vi "SLSC Add Channel Features.vi"(4 "Cluster Enum":T2, 5 "Documentation":string, 6 "description-en":string, 7 "SLSCChannelPath":string, 8 "error in (no error)":errorcluster, 9 "documentation-en":string, 10 "SLSC Command Name":string, 11 "Channel Ref":T1 format="%.0x") -> (0 "error out":errorcluster, 3 "Channel Ref Out":T1 format="%.0x")   [LabVIEW 2015, in "SLSC CD System Explorer.lvlib"]
doc: "Set the channel properties based on the SLSC information, description and documentation."
uses:
  SLSC CD System Explorer.lvlib
  <vilib>/NI Veristand/Custom Device API/Custom Device Item Ref.ctl
  <vilib>/NI Veristand/Custom Device API/Set Item Property (String).vi
  <vilib>/NI VeriStand/Custom Device API/Custom Device API.lvlib
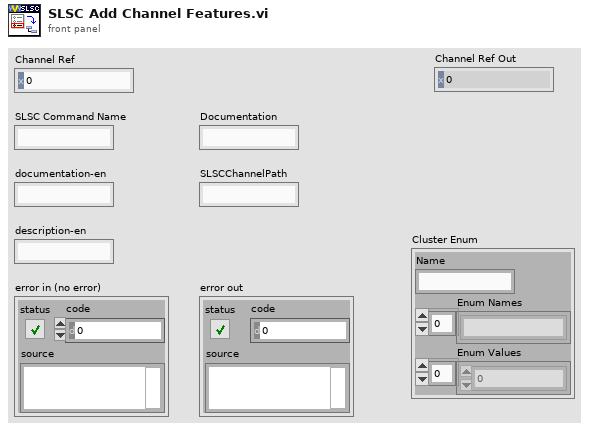
[diagram p1: front panel]
types:
  T1 = typedef "Custom Device API.lvlib/Custom Device Item Ref.ctl" = u64
  T2 = cluster{"Name":string, "Enum Names":string[], "Enum Values":i32[]}
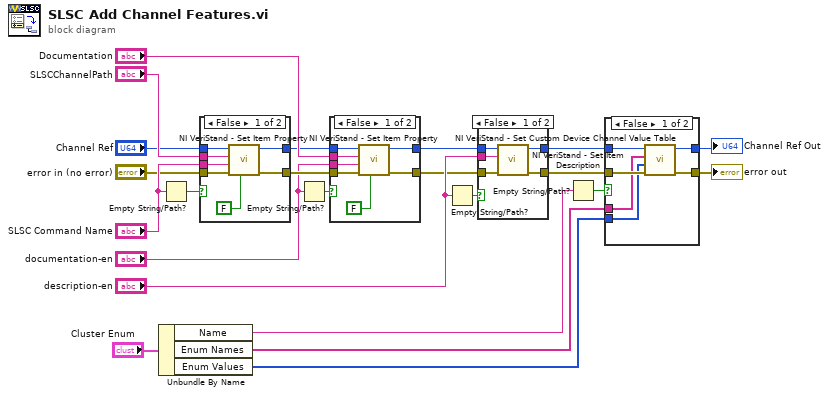
[diagram p0: block diagram]
diagram:
  n1 = Unbundle By Name("Cluster Enum") -> ("Name"=w2:string, "Enum Names"=w4:string[], "Enum Values"=w3:i32[])
  n2 = Empty String/Path?(string/path="SLSC Command Name") -> (empty?=w15:bool)
  n3 = case shown="False" w15 {
    tunnel: "Channel Ref" -> [w30 w32]
    tunnel: "error in (no error)" -> [w29 w31]
    tunnel: [w28 w32] -> w17
    tunnel: [w27 w31] -> w16
    tunnel: "SLSCChannelPath" -> [w26 _]
    tunnel: "SLSC Command Name" -> [w24 _]
    frame False {
      n4 = call-poly <vilib>:"NI VeriStand - Set Item Property.vi"("Binary String (T)"=FALSE, "error in (no error)"=w29, "Value"=w24, "Property Name"=w26, "Item Ref in"=w30) -> ("error out"=w27:errorcluster, "Item Ref out"=w28:T1)  [unwired: 4 in, 1 out]
    }
    frame True {
    }
  }
  n5 = Empty String/Path?(string/path="documentation-en") -> (empty?=w21:bool)
  n6 = case shown="False" w21 {
    tunnel: w17 -> [w39 w41]
    tunnel: w16 -> [w38 w40]
    tunnel: [w37 w41] -> w18
    tunnel: [w36 w40] -> w19
    tunnel: "Documentation" -> [w35 _]
    tunnel: "documentation-en" -> [w33 _]
    frame False {
      n7 = call-poly <vilib>:"NI VeriStand - Set Item Property.vi"("Binary String (T)"=FALSE, "error in (no error)"=w38, "Value"=w33, "Property Name"=w35, "Item Ref in"=w39) -> ("error out"=w36:errorcluster, "Item Ref out"=w37:T1)  [unwired: 4 in, 1 out]
    }
    frame True {
    }
  }
  n8 = Empty String/Path?(string/path="description-en") -> (empty?=w23:bool)
  n9 = case shown="False" w23 {
    tunnel: [w46 w48] -> w8
    tunnel: "description-en" -> [w45 _]
    tunnel: w18 -> [w44 w47]
    tunnel: w19 -> [w43 w48]
    tunnel: [w42 w47] -> w7
    frame False {
      n10 = call <vilib>:"NI VeriStand - Set Item Description.vi"("error in (no error)"=w43, "Description"=w45, "Item Ref in"=w44) -> ("error out"=w46:errorcluster, "Item Ref out"=w42:T1)  [unwired: 6 in, 1 out]
    }
    frame True {
    }
  }
  n11 = Empty String/Path?(string/path=w2) -> (empty?=w9:bool)
  n12 = case shown="False" w9 {
    tunnel: w7 -> [w54 w55]
    tunnel: w8 -> [w53 w56]
    tunnel: [w52 w56] -> w6
    tunnel: w3 -> [w51 _]
    tunnel: w4 -> [w50 _]
    tunnel: [w49 w55] -> w1
    frame False {
      n13 = call <vilib>:"NI VeriStand - Set Custom Device Channel Value Table.vi"("error in (no error)"=w53, "Values"=w51, "Names"=w50, "Channel Ref in"=w54) -> ("error out"=w52:errorcluster, "Channel Ref out"=w49:T1)  [unwired: 6 in]
    }
    frame True {
    }
  }
  "error out" <- w6
  "Channel Ref Out" <- w1
